vi "AutoCad Draw box.vi"(6 "AutoCADFileName":string, 8 "error in (no error)":errorcluster, 9 "Command":string="box 2 3 4\n_-view\n_swiso\n_shademode \n", 11 "open new instance":bool) -> (0 "error out (no error)":errorcluster)   [LabVIEW 2015, in "AguaClara Library.lvlib"]
doc: "Opens a Mathcad Application. \n\nInputs\n\nVisible - If true then the Mathcad Application User Interface is visible.\nOpen New Instance- If true opens a new instance of the Application, otherwise returns a reference to the one open. If false and no Mathcad Applications are running, opens a new reference.\n\nOutputs\n\nIMathcadApp Ref- Reference to the Mathcad Application Class"
uses:
  AguaClara Library.lvlib
panel:
  in  "AutoCAD.IAcadApplication":refnum<k7>
  # "This program opens AutoCAD, opens a file called junk, and draws a box and displays it."
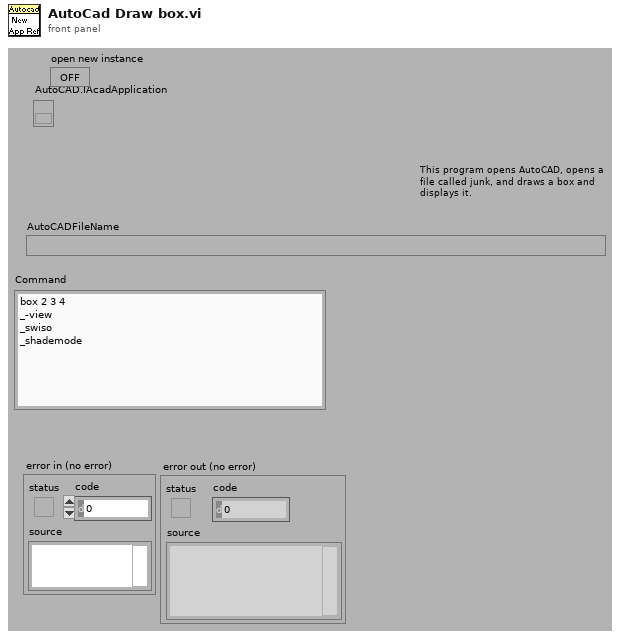
[diagram p1: front panel]
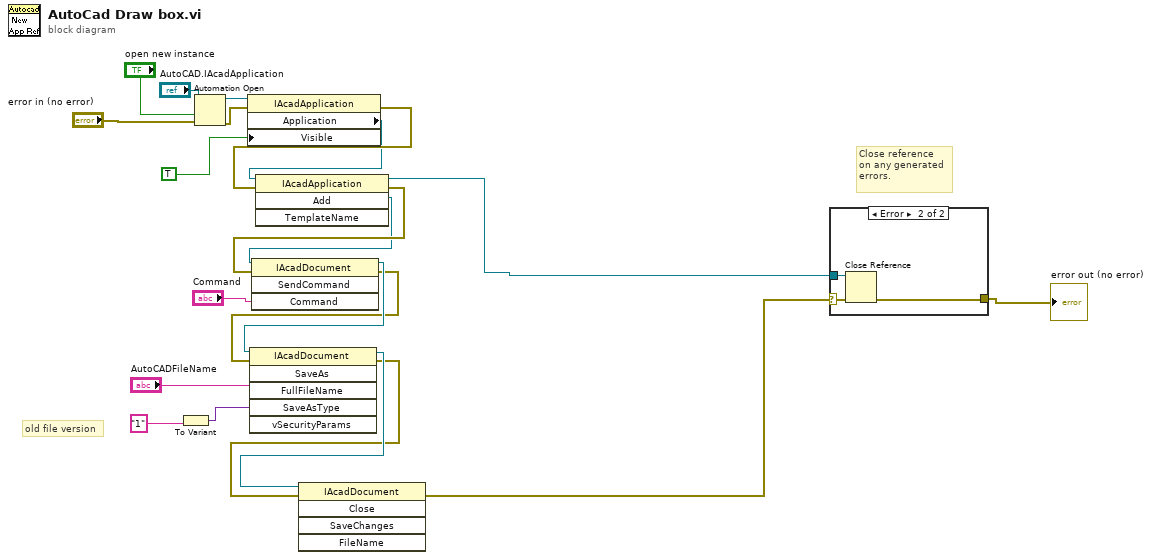
[diagram p0: block diagram]
diagram:
  # "old file version"
  # "Close reference\non any generated\nerrors."
  n1 = To Variant(anything="1") -> (Variant=w2:variant)
  n2 = Automation Open(error in (no error)="error in (no error)", Automation Refnum="AutoCAD.IAcadApplication", 9:"open new instance") -> (Automation Refnum=w16:refnum<k7>, error out=w17:errorcluster)  [unwired: 1 in]
  n3 = property class="IAcadApplication"(reference=w16, error in=w17, "Visible"=TRUE) -> (error out=w8:errorcluster, "Application"=w1:refnum<k7>)  [unwired: 1 out]
  n4 = invoke class="IAcadApplication" method="Add"(reference=w1, error in=w8) -> (reference out=w5:refnum<k7>, error out=w7:errorcluster, "Add"=w6:refnum<k7>)  [unwired: 2 in, 1 out]
  n5 = invoke class="IAcadDocument" method="SendCommand"(reference=w6, error in=w7, "Command"="Command") -> (reference out=w14:refnum<k7>, error out=w13:errorcluster)  [unwired: 1 in, 2 out]
  n6 = invoke class="IAcadDocument" method="SaveAs"(reference=w14, error in=w13, "FullFileName"="AutoCADFileName", "SaveAsType"=w2) -> (reference out=w11:refnum<k7>, error out=w10:errorcluster)  [unwired: 2 in, 4 out]
  n7 = invoke class="IAcadDocument" method="Close"(reference=w11, error in=w10) -> (error out=w9:errorcluster)  [unwired: 3 in, 4 out]
  n8 = case shown="Error" w9 {
    selector: w9 -> [w22 w23]
    tunnel: w5 -> [_ w25]
    tunnel: [w22 w24] -> w21
    frame No Error {
    }
    frame Error {
      n9 = Close Reference(reference=w25, error in (no error)=w23) -> (error out=w24:errorcluster)
    }
  }
  "error out (no error)" <- w21
